vi "I2C Set Clock High.vi"(8 "error in (no error)":errorcluster, 11 "Task In":refnum<k21>) -> (0 "error out":errorcluster, 3 "Task Out":refnum<k21>)   [LabVIEW 2017, in "I2C.lvlib"]
doc: "Sets clock line high."
uses:
  <vilib>/robotics/Protocols/I2C/DAQmx/I2C.lvlib
  <vilib>/DAQmx/read.llb/DAQmx Read (Digital Bool 1Line 1Point).vi
  <vilib>/DAQmx/miscellaneous.llb/DAQmx Fill In Error Info.vi
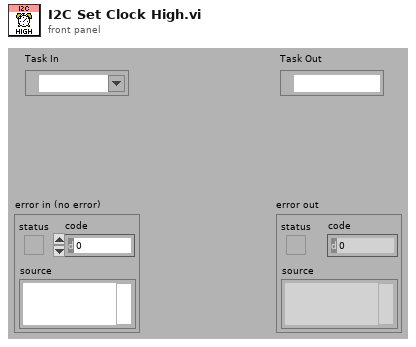
[diagram p1: front panel]
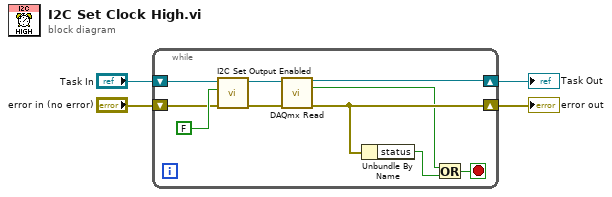
[diagram p0: block diagram]
diagram:
  n1 = while {
    shift-right: [w11] -> w1
    shift-left: "error in (no error)" -> [w6]
    shift-right: [w5] -> w2
    shift-left: "Task In" -> [w14]
    stop <- w8 stop-if-true
    n2 = call <vilib>:"I2C Set Output Enabled.vi"("error in (no error)"=w6, "Output Enabled (T:Enable)"=FALSE ("DO.Tristate"), "Task In"=w14) -> ("error out"=w12:errorcluster, "Task Out"=w13:refnum<k21>)  [unwired: 7 in]
    n3 = call-poly <vilib>:"DAQmx Read.vi"("task/channels in"=w13, "error in"=w12) -> ("task out"=w5:refnum<k21>, "data"=w9:bool, "error out"=w11:errorcluster)  [unwired: 11 in]
    n4 = Unbundle By Name(w11) -> ("status"=w10:bool)
    n5 = Or(x=w9, y=w10) -> (x .or. y?=w8:bool)
  }
  "error out" <- w1
  "Task Out" <- w2
